vi "Execute.vi"(8 "error in":errorcluster, 9 "Consumer Queues in":T1, 10 "DAC Process Command in":refnum<class "Select DAC Config File.lvclass">, 11 "DAC Process Data in":T2) -> (0 "error out":errorcluster, 1 "Consumer Queues out":T1, 2 "Stop?":bool, 3 "DAC Process Data out":T2)   [LabVIEW 2019, in "DAC Process.lvlib" / "Select DAC Config File.lvclass"]
uses:
  Select DAC Config File.lvclass
  C:/Users/wg/Documents/LV_Projects/test-stand/App/DAC Process/Generic DAC Command/Generic DAC Process Command.lvclass
  DAC Process Data.ctl
  Generic Test Stand/Generic Test Stand.lvclass
  TS Framework/ExeLogging/DAC Logger/DAC Logger.lvclass
  DAC State.ctl
  TS Framework/Consumer Queues.ctl
  UI Process/Generic UI Command/Generic UI Process Command.lvclass
  Generic DAC Command/Generic DAC Process Command.lvclass
  Trig Process/Generic Trig Command/Generic Trig Process Command.lvclass
  Generic Test Stand/Generic Test Stand.lvclass/Generic Test Stand.ctl
  UI Process/Update UI Status/Update UI Status.lvclass
  Configure DAC Test Stand/Configure DAC Test Stand.lvclass
  UI Process/Update UI Status/Update UI Status.lvclass/Update UI Status.ctl
  Generic DAC Command/Generic DAC Process Command.lvclass/Generic DAC Process Command.ctl
  C:/Users/wg/Documents/LV_Projects/test-stand/App/Generic Command/Generic Command.lvclass
  DAC Process.lvlib
  TS Framework/TS Framework.lvlib
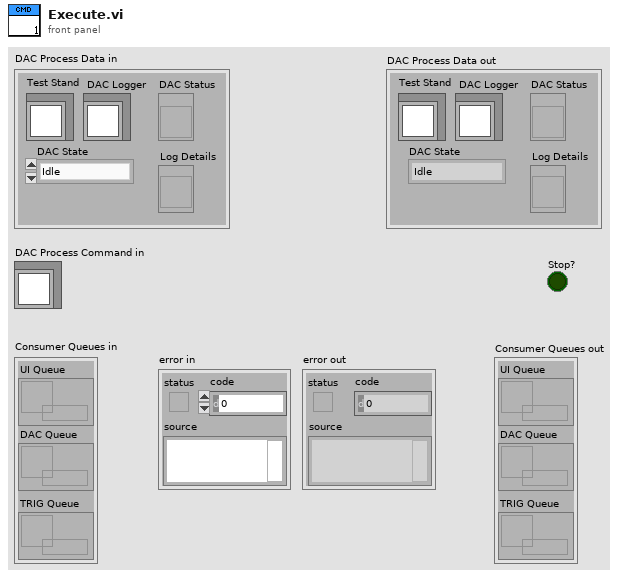
[diagram p1: front panel]
types:
  T1 = typedef "TS Framework.lvlib/Consumer Queues.ctl" = cluster{"UI Queue":refnum<queue>, "DAC Queue":refnum<queue>, "TRIG Queue":refnum<queue>}
  T2 = typedef "DAC Process.lvlib/DAC Process Data.ctl" = cluster{"Test Stand":refnum<class "Generic Test Stand.lvclass">, " DAC Logger":refnum<class "DAC Logger.lvclass">, "DAC State":T3, "DAC Status":refnum<vi>, "Log Details":refnum<vi>}
  T3 = typedef "DAC Process.lvlib/DAC State.ctl" = enum16{"Idle", "Acquiring"}
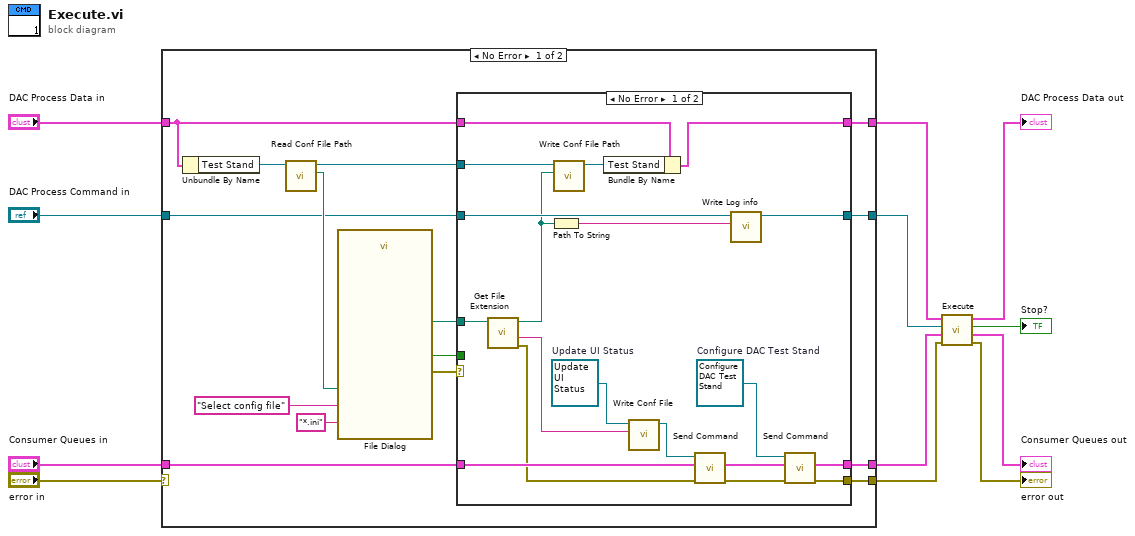
[diagram p0: block diagram]
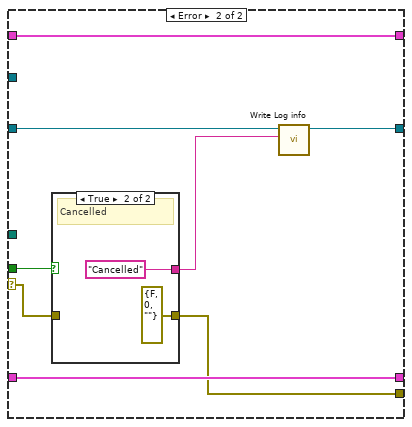
[diagram p2: hidden frame]
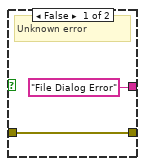
[diagram p3: hidden frame]
diagram:
  n1 = case shown="No Error" "error in" {
    selector: "error in" -> [_ w62]
    tunnel: "DAC Process Data in" -> [w20 w60]
    tunnel: "Consumer Queues in" -> [w15 w61]
    tunnel: [w18 w62] -> w3
    tunnel: [w17 w61] -> w4
    tunnel: [w19 w60] -> w5
    tunnel: "DAC Process Command in" -> [w14 w59]
    tunnel: [w13 w59] -> w1
    frame No Error {
      n2 = Unbundle By Name(w20) -> ("Test Stand"=w27:refnum<class "Generic Test Stand.lvclass">)
      n3 = call "Read Conf File Path.vi"("Generic Test Stand in"=w27) -> ("Conf File Path"=w21:path, "Generic Test Stand out"=w16:refnum<class "Generic Test Stand.lvclass">)  [unwired: 8 in, 1 out]
      n4 = call "File Dialog"("start path"=w21, "prompt"="Select config file", "pattern (all files)"="*.ini") -> ("selected path"=w22:path, "cancelled"=w23:bool, "error out"=w24:errorcluster)  [unwired: 9 in, 1 out]
      n5 = case shown="No Error" w24 {
        selector: w24 -> [_ w48]
        tunnel: w22 -> [w46 _]
        tunnel: w23 -> [_ w54]
        tunnel: w20 -> [w45 w50]
        tunnel: [w43 w50] -> w19
        tunnel: [w33 w47] -> w18
        tunnel: [w34 w49] -> w17
        tunnel: w16 -> [w40 _]
        tunnel: w15 -> [w38 w49]
        tunnel: w14 -> [w31 w53]
        tunnel: [w30 w52] -> w13
        frame No Error {
          w32 = refnum<class "Configure DAC Test Stand.lvclass"> refnum  # Configure DAC Test Stand
          w41 = refnum<class "Update UI Status.lvclass"> refnum  # Update UI Status
          n6 = call <vilib>:"Get File Extension.vi"("file"=w46) -> ("error out"=w37:errorcluster, "filename without extension"=w39:string, "dup file"=w29:path)  [unwired: 6 in, 2 out]
          n7 = Path To String(path=w29) -> (string=w28:string)
          n8 = call "Write Conf File Path.vi"("Conf File Path"=w29, "Generic Test Stand in"=w40) -> ("Generic Test Stand out"=w44:refnum<class "Generic Test Stand.lvclass">)  [unwired: 8 in, 1 out]
          n9 = Bundle By Name(cluster=w45, "Test Stand"=w44) -> (w43:T2)
          n10 = call "Write Conf File.vi"("Conf File"=w39, "Update UI Status in"=w41) -> ("Update UI Status out"=w42:refnum<class "Update UI Status.lvclass">)  [unwired: 9 in]
          n11 = call-dynamic "Send Command.vi"("error in (no error)"=w37, "Consumer Queues in"=w38, "UI Process Command in"=w42) -> ("error out"=w35:errorcluster, "Consumer Queues out"=w36:T1)  [unwired: 7 in]
          n12 = call "Write Log info.vi"("Log info"=w28, "Generic DAC Process Command in"=w31) -> ("Generic DAC Process Command out"=w30:refnum<class "Select DAC Config File.lvclass">)  [unwired: 9 in]
          n13 = call-dynamic "Send Command.vi"("error in (no error)"=w35, "Consumer Queues in"=w36, "DAC Process Command"=w32) -> ("error out"=w33:errorcluster, "Consumer Queues out"=w34:T1)  [unwired: 7 in]
        }
        frame Error {
          n14 = case shown="True" w54 {
            tunnel: ["File Dialog Error" "Cancelled"] -> w51
            tunnel: w48 -> [w55 _]
            tunnel: [w55 errorcluster {"status"=FALSE, "code"=0, "source"=""} ("error IO")] -> w47
            frame False {
              # "Unknown error"
            }
            frame True {
              # "Cancelled"
            }
          }
          n15 = call "Write Log info.vi"("Log info"=w51, "Generic DAC Process Command in"=w53) -> ("Generic DAC Process Command out"=w52:refnum<class "Select DAC Config File.lvclass">)  [unwired: 9 in]
        }
      }
    }
    frame Error {
    }
  }
  n16 = call-parent "Execute.vi"("error in"=w3, "Consumer Queues in"=w4, "DAC Process Command in"=w1, "DAC Process Data in"=w5) -> ("error out"=→"error out":errorcluster, "Consumer Queues out"=→"Consumer Queues out":T1, "Stop?"=→"Stop?":bool, "DAC Process Data out"=→"DAC Process Data out":T2)  [unwired: 4 in]
